vi "Leftable.vi"(1 "方块":dbl[][](array[numeric]), 2 "x":dbl) -> (0 "输出":bool)   [LabVIEW 2016]
panel:
  out "数值":dbl
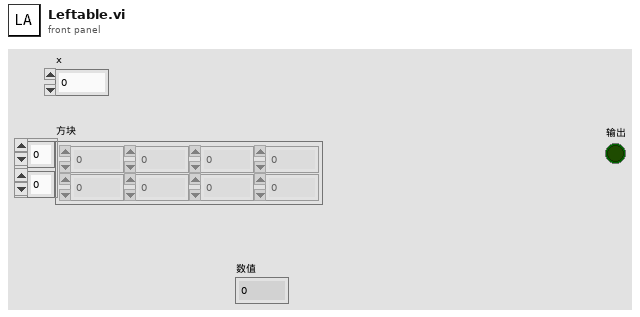
[diagram p1: front panel]
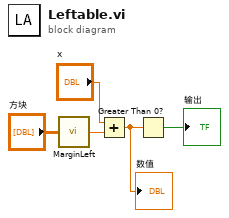
[diagram p0: block diagram]
diagram:
  n1 = call "MarginLeft.vi"("输入"="方块") -> ("输出"=w2:dbl)
  n2 = Add(x="x", y=w2) -> (x+y=w1:dbl)
  "数值" <- w1
  n3 = Greater Than 0?(x=w1) -> (x > 0?=→"输出":bool)
